vi "Marker Data_RageATE.vi"(0 "VISA resource name":refnum<visa-resource-name>, 1 "Channel (1)":i32=1, 2 "Trace (1)":i32=1, 3 "Marker (1)":i32=1, 11 "error in (no error)":errorcluster) -> (4 "VISA resource name out":refnum<visa-resource-name>, 6 "X Value":dbl format="%^.2e", 10 "Y Real Value":dbl format="%^.2e", 14 "Y Imaginary Value":dbl format="%^.2e", 15 "error out":errorcluster)   [LabVIEW 2018, in "Agilent ENA Series.lvlib"]
doc: "Reads out the response value of selected marker, for the active trace of selected channel.\n\nNote:\nWhen the reference marker mode is enabled, the readout value is the value relative to the reference marker."
uses:
  Agilent ENA Series.lvlib
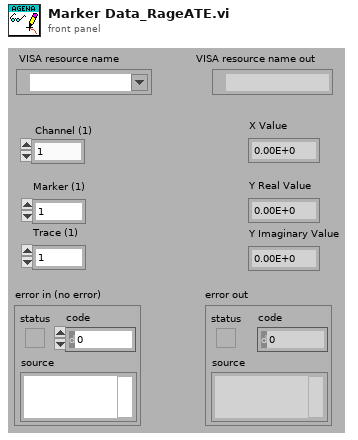
[diagram p1: front panel]
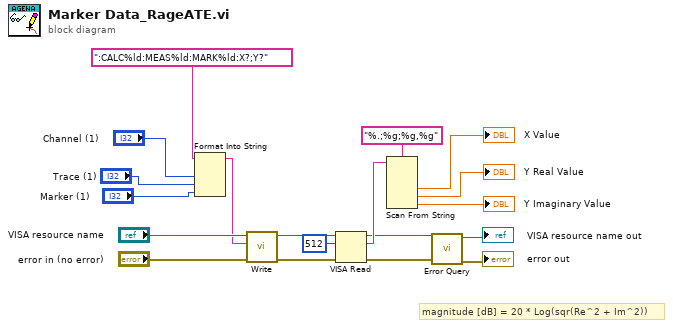
[diagram p0: block diagram]
diagram:
  # "magnitude [dB] = 20 * Log(sqr(Re^2 + Im^2))"
  n1 = Format Into String(format string=":CALC%ld:MEAS%ld:MARK%ld:X?;Y?", "Channel (1)", "Trace (1)", "Marker (1)") -> (resulting string=w10:string)  [unwired: 2 in, 1 out]
  n2 = call "Write.vi"("error in (no error)"="error in (no error)", "String ()"=w10, "VISA resource name"="VISA resource name") -> ("error out"=w16:errorcluster, "VISA resource name out"=w17:refnum<visa-resource-name>)  [unwired: 6 in, 1 out]
  n3 = VISA Read(VISA resource name=w17, byte count=u32 512, error in (no error)=w16) -> (VISA resource name out=w9:refnum<visa-resource-name>, read buffer=w14:string, error out=w8:errorcluster)  [unwired: 1 out]
  n4 = Scan From String(format string="%.;%g;%g,%g", input string=w14) -> (output 1=→"X Value":dbl, output 2=→"Y Real Value":dbl, output 3=→"Y Imaginary Value":dbl)  [unwired: 5 in, 3 out]
  n5 = call "Error Query.vi"("error in (no error)"=w8, "VISA resource name"=w9) -> ("error out"=→"error out":errorcluster, "VISA resource name out"=→"VISA resource name out":refnum<visa-resource-name>)  [unwired: 6 in, 2 out]
